vi "Motor-HandPaddle.vi"(1 "Motor":string) -> ()   [LabVIEW 2009]
uses:
  Ressources/StopUserEvent.ctl
  Ressources/Stop.ctl
panel:
  out "Position":i32
  in  "Step Size":i32(slide) scale=0.0..100.0
  in  "stop":bool
  in  ">":bool
  in  "<":bool
  out "Stop User Event":T1
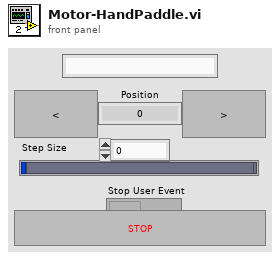
[diagram p1: front panel]
types:
  T1 = typedef "StopUserEvent.ctl" = refnum<user-event>
  T2 = typedef "Stop.ctl" = bool
  T3 = typedef "MotorStatus.ctl" = cluster{"Managed?":bool, "Position":i32, "Name":string, "Status":enum16{"OFF", "IDLE", "MOVING", "HOMING"}}
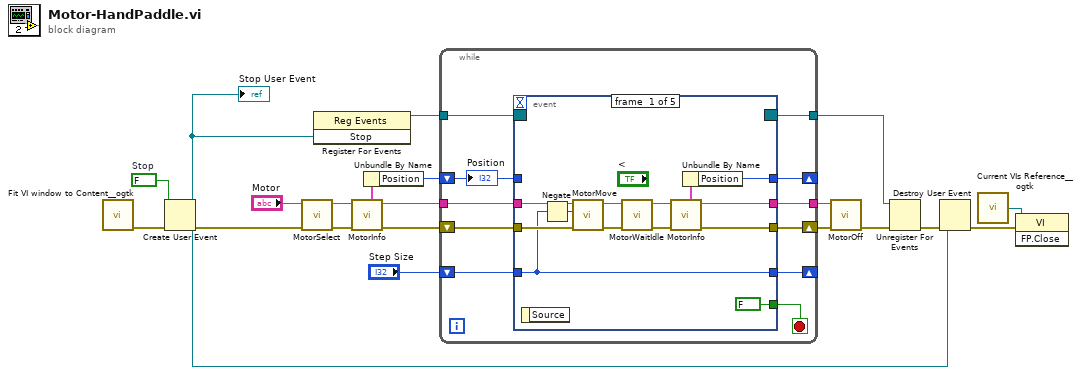
[diagram p0: block diagram]
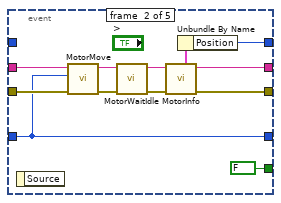
[diagram p2: hidden frame]
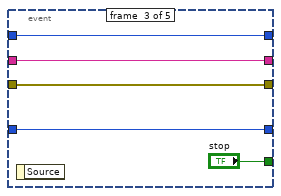
[diagram p3: hidden frame]
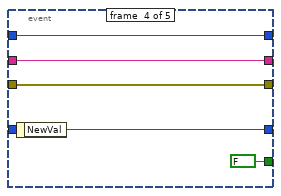
[diagram p4: hidden frame]
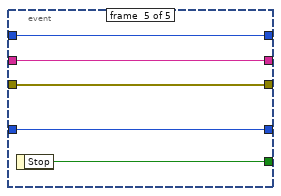
[diagram p5: hidden frame]
diagram:
  w3 = T2 FALSE  # Stop
  n1 = call <userlib>:"Fit VI window to Content__ogtk.vi"() -> ("error out"=w4:errorcluster)  [unwired: 3 in, 4 out]
  n2 = Create User Event(user event datatype=w3, error in=w4) -> (user event=w1:refnum<user-event>, error out=w2:errorcluster)
  "Stop User Event" <- w1
  n3 = call "MotorSelect.vi"("Motor"="Motor", "error in (no error)"=w2) -> ("Motor out"=w17:string, "error out"=w18:errorcluster)  [unwired: 6 out]
  n4 = register-events(w1) -> (reference out=w10:refnum<event-registration>)  [unwired: 2 in, 1 out]
  n5 = call "MotorInfo.vi"("error in (no error)"=w18, "Motor"=w17) -> ("error out"=w15:errorcluster, "Motor out"=w16:string, "Axis status"=w14:T3)  [unwired: 5 out]
  n6 = Unbundle By Name(w14) -> ("Position"=w13:i32)
  n7 = while {
    shift-right: [w29] -> w12
    shift-left: w15 -> [w31]
    tunnel: w16 -> [w30]
    tunnel: [w28] -> w11
    shift-right: [w26] -> _
    shift-left: "Step Size" -> [w27]
    shift-right: [w25] -> _
    shift-left: w13 -> [w24]
    tunnel: w10 -> [w22]
    tunnel: [w21] -> w8
    stop <- w23 stop-if-true
    n8 = event shown="[4] <Stop>: User Event" {
      selector: w22 -> [_ _ _ _ _]
      dyn-events: [_ _ _ _ _] -> w21
      timeout: _ -> [_ _ _ _ _]
      tunnel: w31 -> [w44 w54 w59 w64 w68]
      tunnel: w30 -> [w42 w53 w60 w65 w67]
      tunnel: [w34 w48 w59 w64 w68] -> w29
      tunnel: [w35 w47 w60 w65 w67] -> w28
      tunnel: w27 -> [w40 w52 w58 _ w69]
      tunnel: [w40 w52 w58 w66 w69] -> w26
      tunnel: [w33 w46 w61 w63 w70] -> w25
      tunnel: w24 -> [_ _ w61 w63 w70]
      tunnel: [FALSE ("stop") FALSE ("stop") "stop" FALSE ("stop") w71] -> w23
      event #0 {
        n9 = event-data() -> ()  [unwired: 2 out]
        n10 = Negate(x=w40) -> (-x=w39:i32)
        n11 = call "MotorMove.vi"("Motor"=w42, "Movement"=w39, "error in (no error)"=w44) -> ("Motor out"=w41:string, "error out"=w43:errorcluster)  [unwired: 5 out]
        n12 = call "MotorWaitIdle.vi"("Motor"=w41, "error in (no error)"=w43) -> ("Motor out"=w37:string, "error out"=w36:errorcluster)  [unwired: 6 out]
        n13 = call "MotorInfo.vi"("error in (no error)"=w36, "Motor"=w37) -> ("error out"=w34:errorcluster, "Motor out"=w35:string, "Axis status"=w38:T3)  [unwired: 5 out]
        n14 = Unbundle By Name(w38) -> ("Position"=w33:i32)
      }
      event #1 {
        n15 = event-data() -> ()  [unwired: 2 out]
        n16 = call "MotorMove.vi"("Motor"=w53, "Movement"=w52, "error in (no error)"=w54) -> ("Motor out"=w55:string, "error out"=w56:errorcluster)  [unwired: 5 out]
        n17 = call "MotorWaitIdle.vi"("Motor"=w55, "error in (no error)"=w56) -> ("Motor out"=w50:string, "error out"=w49:errorcluster)  [unwired: 6 out]
        n18 = call "MotorInfo.vi"("error in (no error)"=w49, "Motor"=w50) -> ("error out"=w48:errorcluster, "Motor out"=w47:string, "Axis status"=w51:T3)  [unwired: 5 out]
        n19 = Unbundle By Name(w51) -> ("Position"=w46:i32)
      }
      event #2 {
        n20 = event-data() -> ()  [unwired: 2 out]
      }
      event #3 {
        n21 = event-data() -> ("NewVal"=w66:i32)  [unwired: 1 out]
      }
      event #4 {
        n22 = event-data() -> ("Stop"=w71:T2)  [unwired: 1 out]
      }
    }
    "Position" <- w24
  }
  n23 = call "MotorOff.vi"("Motor"=w11, "error in (no error)"=w12) -> ("error out"=w9:errorcluster)  [unwired: 7 out]
  n24 = Unregister For Events(event registration refnum=w8, error in=w9) -> (error out=w7:errorcluster)
  n25 = Destroy User Event(user event=w1, error in=w7) -> (error out=w6:errorcluster)
  n26 = call <userlib>:"Current VIs Reference__ogtk.vi"() -> ("Current VI's reference"=w5:refnum<vi>)  [unwired: 5 out]
  n27 = invoke class="VI" method="FP.Close"(reference=w5, error in=w6) -> ()  [unwired: 1 in, 3 out]
